vi "zurich_lock_in_Manage_Monitor.vi"(3 "Lockin # (in)":i32, 4 "System Monitor Variables (in)":T2, 5 "Command (in)":T1, 6 "Global Status (in)":T1, 7 "queue (in)":refnum<queue>) -> (0 "Monitor (out)":T1, 1 "System Monitor Variables (out)":T2)   [LabVIEW 2019]
uses:
  Global/Global Variables/System Monitor Cluster.ctl
  zurich_lock_in/zurichinstMonitor.ctl
  Instrument_Setup.vi
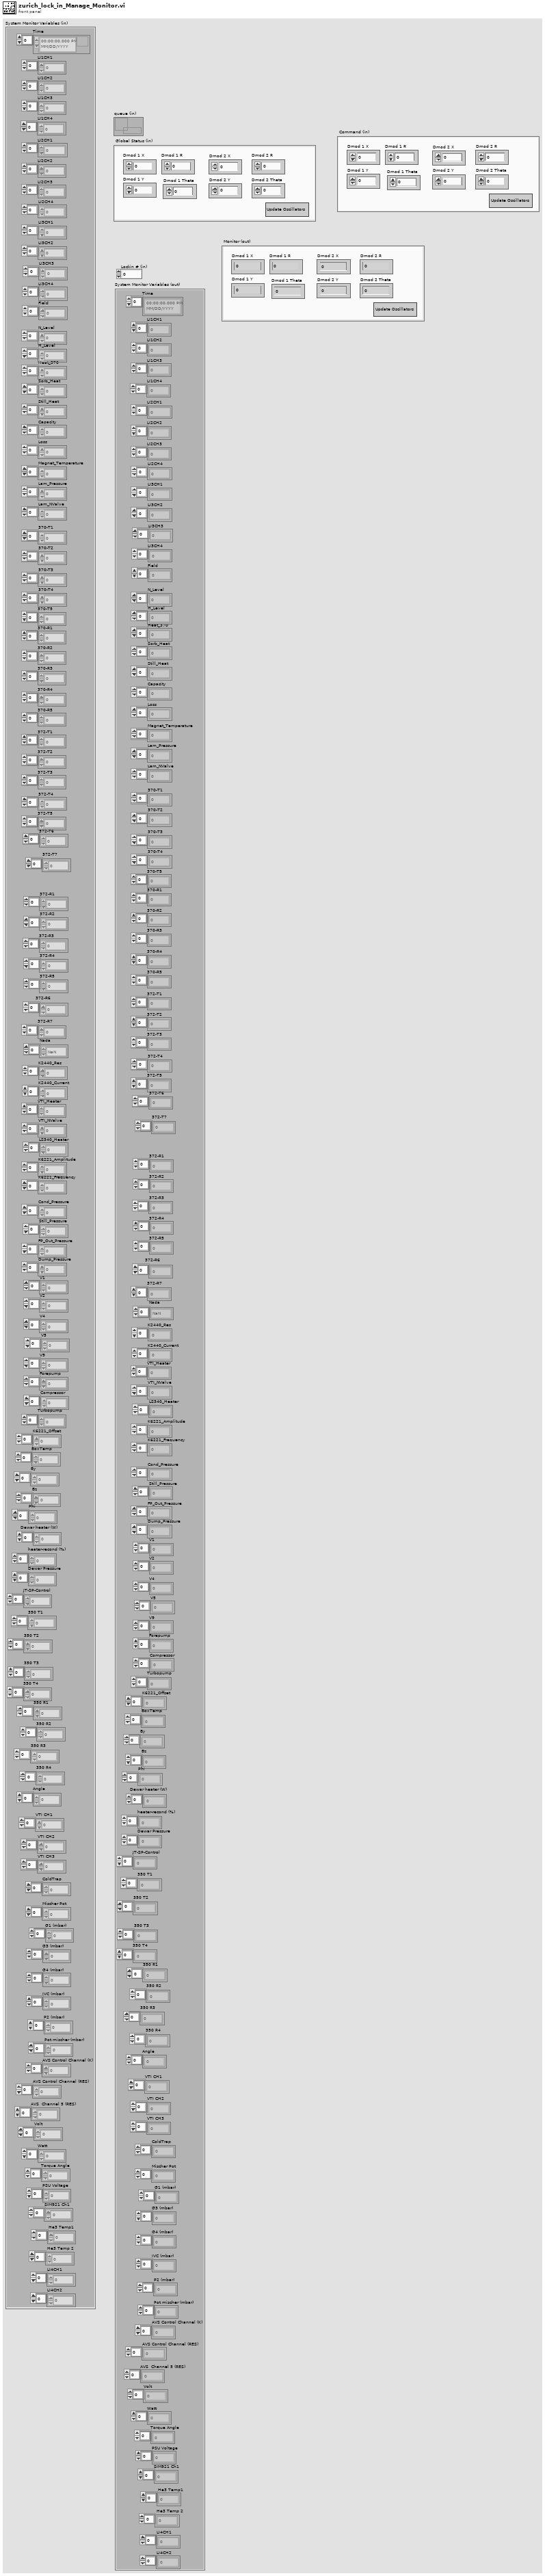
[diagram p1: front panel]
types:
  T1 = typedef "zurichinstMonitor.ctl" = cluster{"Dmod 1 X":dbl, "Dmod 1 Y":dbl, "Dmod 1 R":dbl, "Dmod 1 Theta":dbl, "Update Oscillators":bool, "Dmod 2 X":dbl, "Dmod 2 R":dbl, "Dmod 2 Y":dbl, "Dmod 2 Theta":dbl}
  T2 = typedef "System Monitor Cluster.ctl" = cluster{"Time":timestamp[], "LI1CH1":dbl[], "LI1CH2":dbl[], "LI2CH1":dbl[], "LI2CH2":dbl[], "LI3CH1":dbl[], "LI3CH2":dbl[], "Field":dbl[], "N_Level":dbl[], "H_Level":dbl[], "Heat_370":dbl[], "Sorb_Heat":dbl[], "Still_Heat":dbl[], "Capacity":dbl[], "Loss":dbl[], "Magnet_Temperature":dbl[], "Lam_Pressure":dbl[], "Lam_NValve":dbl[], "370-T1":dbl[], "370-T2":dbl[], "370-T3":dbl[], "370-T4":dbl[], "370-T5":dbl[], "370-R1":dbl[], "370-R2":dbl[], "370-R3":dbl[], "370-R4":dbl[], "370-R5":dbl[], "372-T1":dbl[], "372-T2":dbl[], "372-T3":dbl[], "372-T4":dbl[], "372-T5":dbl[], "372-T6":dbl[], "372-R1":dbl[], "372-R2":dbl[], "372-R3":dbl[], "372-R4":dbl[], "372-R5":dbl[], "372-R6":dbl[], "Nada":dbl[], "K2440_Res":dbl[], "K2440_Current":dbl[], "VTI_Heater":dbl[], "VTI_NValve":dbl[], "LS340_Heater":dbl[], "K6221_Amplitude":dbl[], "K6221_Frequency":dbl[], "Cond_Pressure":dbl[], "Still_Pressure":dbl[], "FP_Out_Pressure":dbl[], "Dump_Pressure":dbl[], "V1":dbl[], "V2":dbl[], "V4":dbl[], "V5":dbl[], "V9":dbl[], "Forepump":dbl[], "Compressor":dbl[], "K6221_Offset":dbl[], "BoxTemp":dbl[], "By":dbl[], "Bz":dbl[], "Phi":dbl[], "heater-recond (%)":dbl[], "Dewar Pressure ":dbl[], "JT-SP-Control":dbl[], "350 T1":dbl[], "350 T2":dbl[], "350 T3":dbl[], "350 T4":dbl[], "350 R1":dbl[], "350 R2":dbl[], "350 R3":dbl[], "350 R4":dbl[], "Angle":dbl[], "VTI CH1":dbl[], "VTI CH2":dbl[], "VTI CH3":dbl[], "ColdTrap":dbl[], "Mischer Pot":dbl[], "G1 (mbar)":dbl[], "G3 (mbar) ":dbl[], "G4 (mbar)":dbl[], "IVC (mbar)":dbl[], "P2 (mbar) ":dbl[], "Pot mischer (mbar)":dbl[], "AVS Control Channel (K)":dbl[], "AVS Control Channel (RES)":dbl[], "AVS  Channel 5 (RES) ":dbl[], "LI3CH3":dbl[], "LI3CH4":dbl[], "LI1CH3":dbl[], "LI1CH4":dbl[], "LI2CH3":dbl[], "LI2CH4":dbl[], "Volt":dbl[], "Watt":dbl[], "Torque Angle":dbl[], "Dewar heater (W)":dbl[], "PSU Voltage":dbl[], "Turbopump":dbl[], "372-R7":dbl[], "372-T7":dbl[], "SIM921 Ch1":dbl[], " He3 Temp1":dbl[], " He3 Temp 2":dbl[], "LI4CH1":dbl[], "LI4CH2":dbl[]}
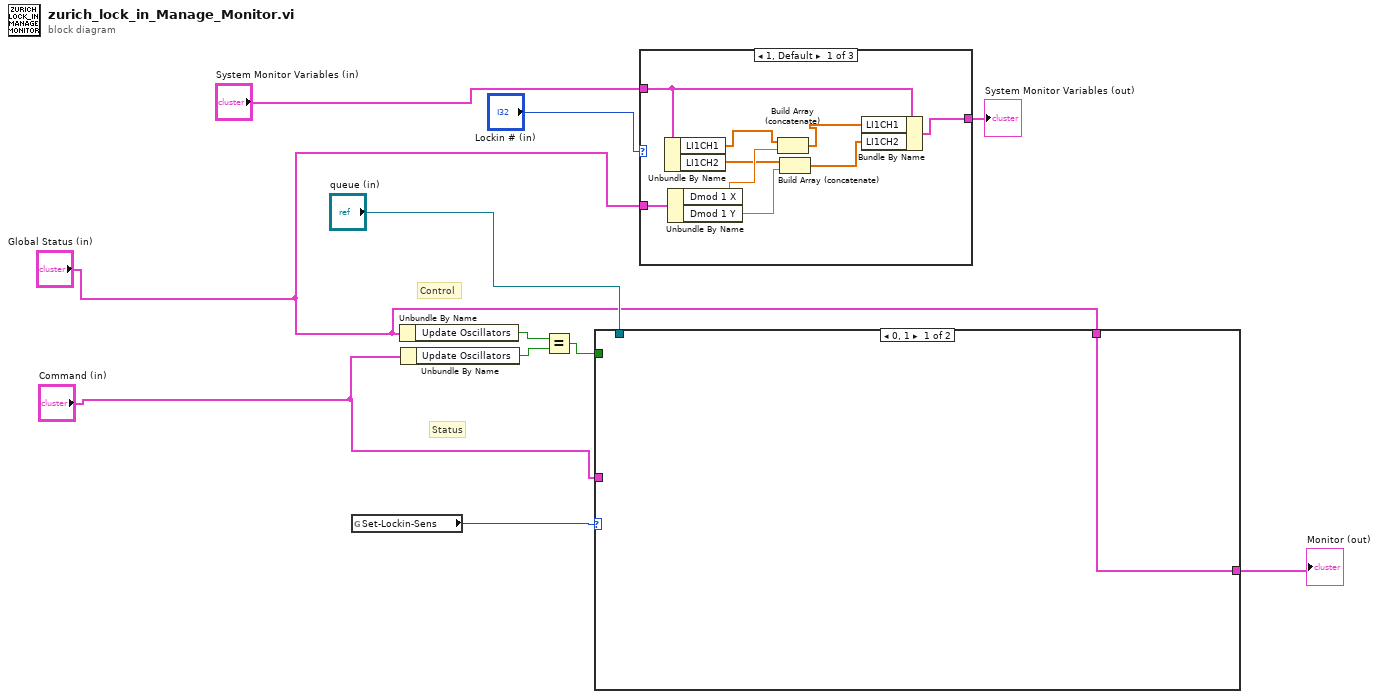
[diagram p0: block diagram]
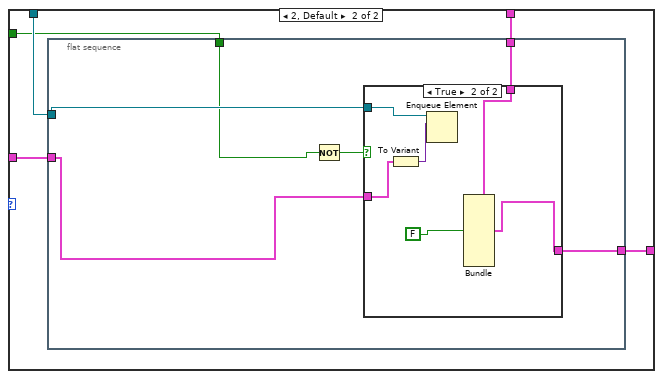
[diagram p2: hidden frame]
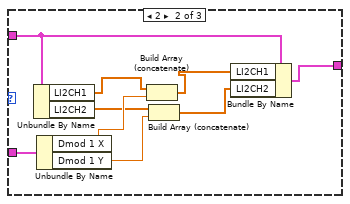
[diagram p4: hidden frame]
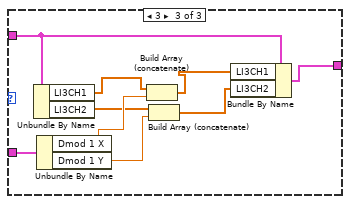
[diagram p5: hidden frame]
diagram:
  # "Status"
  # "Control"
  n1 = global read "Instrument_Setup.vi" "Set-Lockin-Sens"() -> (w4:u16)
  n2 = Unbundle By Name("Global Status (in)") -> ("Update Oscillators"=w6:bool)
  n3 = Unbundle By Name("Command (in)") -> ("Update Oscillators"=w5:bool)
  n4 = Equal?(x=w6, y=w5) -> (x = y?=w10:bool)
  n5 = case shown="0, 1" w4 {
    tunnel: "queue (in)" -> [_ w17]
    tunnel: w10 -> [_ w16]
    tunnel: [w12 w15] -> w1
    tunnel: "Command (in)" -> [_ w14]
    tunnel: "Global Status (in)" -> [w12 w13]
    frame 0, 1 {
    }
    frame 2, Default {
      n6 = flat-sequence {
        tunnel: w17 -> [w23]
        tunnel: w14 -> [w20]
        tunnel: [w21] -> w15
        tunnel: w16 -> [w19]
        tunnel: w13 -> [w18]
        frame #0 {
          n7 = Not(x=w19) -> (.not. x?=w22:bool)
          n8 = case shown="True" w22 {
            tunnel: w23 -> [_ w30]
            tunnel: w20 -> [_ w28]
            tunnel: [w24 w25] -> w21
            tunnel: w18 -> [w24 w27]
            frame False {
            }
            frame True {
              n9 = To Variant(anything=w28) -> (Variant=w29:variant)
              n10 = Enqueue Element(queue=w30, element=w29) -> ()  [unwired: 2 in, 3 out]
              n11 = Bundle(cluster=w27, "Update Oscillators"=FALSE) -> (w25:T1)  [unwired: 8 in]
            }
          }
        }
      }
    }
  }
  "Monitor (out)" <- w1
  n12 = case shown="1, Default" "Lockin # (in)" {
    tunnel: "Global Status (in)" -> [w39 w48 w57]
    tunnel: "System Monitor Variables (in)" -> [w38 w47 w56]
    tunnel: [w31 w40 w49] -> w8
    frame 1, Default {
      n13 = Unbundle By Name(w38) -> ("LI1CH1"=w36:dbl[], "LI1CH2"=w34:dbl[])
      n14 = Unbundle By Name(w39) -> ("Dmod 1 X"=w37:dbl, "Dmod 1 Y"=w33:dbl)
      n15 = Build Array (concatenate)(w36, w37) -> (w35:dbl[])
      n16 = Build Array (concatenate)(w34, w33) -> (w32:dbl[])
      n17 = Bundle By Name(cluster=w38, "LI1CH1"=w35, "LI1CH2"=w32) -> (w31:T2)
    }
    frame 2 {
      n18 = Unbundle By Name(w47) -> ("LI2CH1"=w45:dbl[], "LI2CH2"=w43:dbl[])
      n19 = Unbundle By Name(w48) -> ("Dmod 1 X"=w46:dbl, "Dmod 1 Y"=w42:dbl)
      n20 = Build Array (concatenate)(w45, w46) -> (w44:dbl[])
      n21 = Build Array (concatenate)(w43, w42) -> (w41:dbl[])
      n22 = Bundle By Name(cluster=w47, "LI2CH1"=w44, "LI2CH2"=w41) -> (w40:T2)
    }
    frame 3 {
      n23 = Unbundle By Name(w56) -> ("LI3CH1"=w54:dbl[], "LI3CH2"=w52:dbl[])
      n24 = Unbundle By Name(w57) -> ("Dmod 1 X"=w55:dbl, "Dmod 1 Y"=w51:dbl)
      n25 = Build Array (concatenate)(w54, w55) -> (w53:dbl[])
      n26 = Build Array (concatenate)(w52, w51) -> (w50:dbl[])
      n27 = Bundle By Name(cluster=w56, "LI3CH1"=w53, "LI3CH2"=w50) -> (w49:T2)
    }
  }
  "System Monitor Variables (out)" <- w8
